vi "Old Vision Processing.vi"(4 "error in (no error)":errorcluster) -> ()   [LabVIEW 2011]
doc: "This VI runs in parallel to other tasks. It gets images from the camera, processes them for color or shape and use that information to affect robot behavior."
uses:
  Robot Global Data.vi
panel:
  out "deltay":dbl
  out "deltax":dbl
  out "distance":dbl
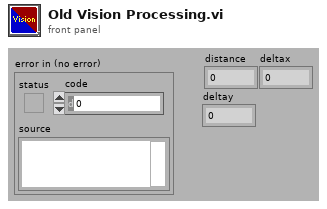
[diagram p1: front panel]
types:
  T1 = typedef "Image Type" = u32
  T2 = typedef "IMAQ Image.ctl" = refnum<image>
  T3 = typedef "WPI_CameraDevRef.ctl" = cluster{"Camera Address":string, "CameraStatus":errorcluster, "Acquire Image Notifier":refnum<notifier>}
  T4 = typedef "WPI_CameraImageSize.ctl" = enum16{"640x480", "320x240", "160x120"}
  T5 = typedef "CAN Data.ctl" = cluster{"Turret Position":dbl, "Turret Elevation":dbl, "Shooter Top Speed":dbl, "Shooter Bottom Speed":dbl}
  T6 = typedef "Position Typedef.ctl" = cluster{"X":dbl, "Y":dbl, "Heading":dbl}
  T7 = typedef "Target Typedef.ctl" = cluster{"X":dbl, "Y":dbl, "Ultrasonic Range (in)":dbl}
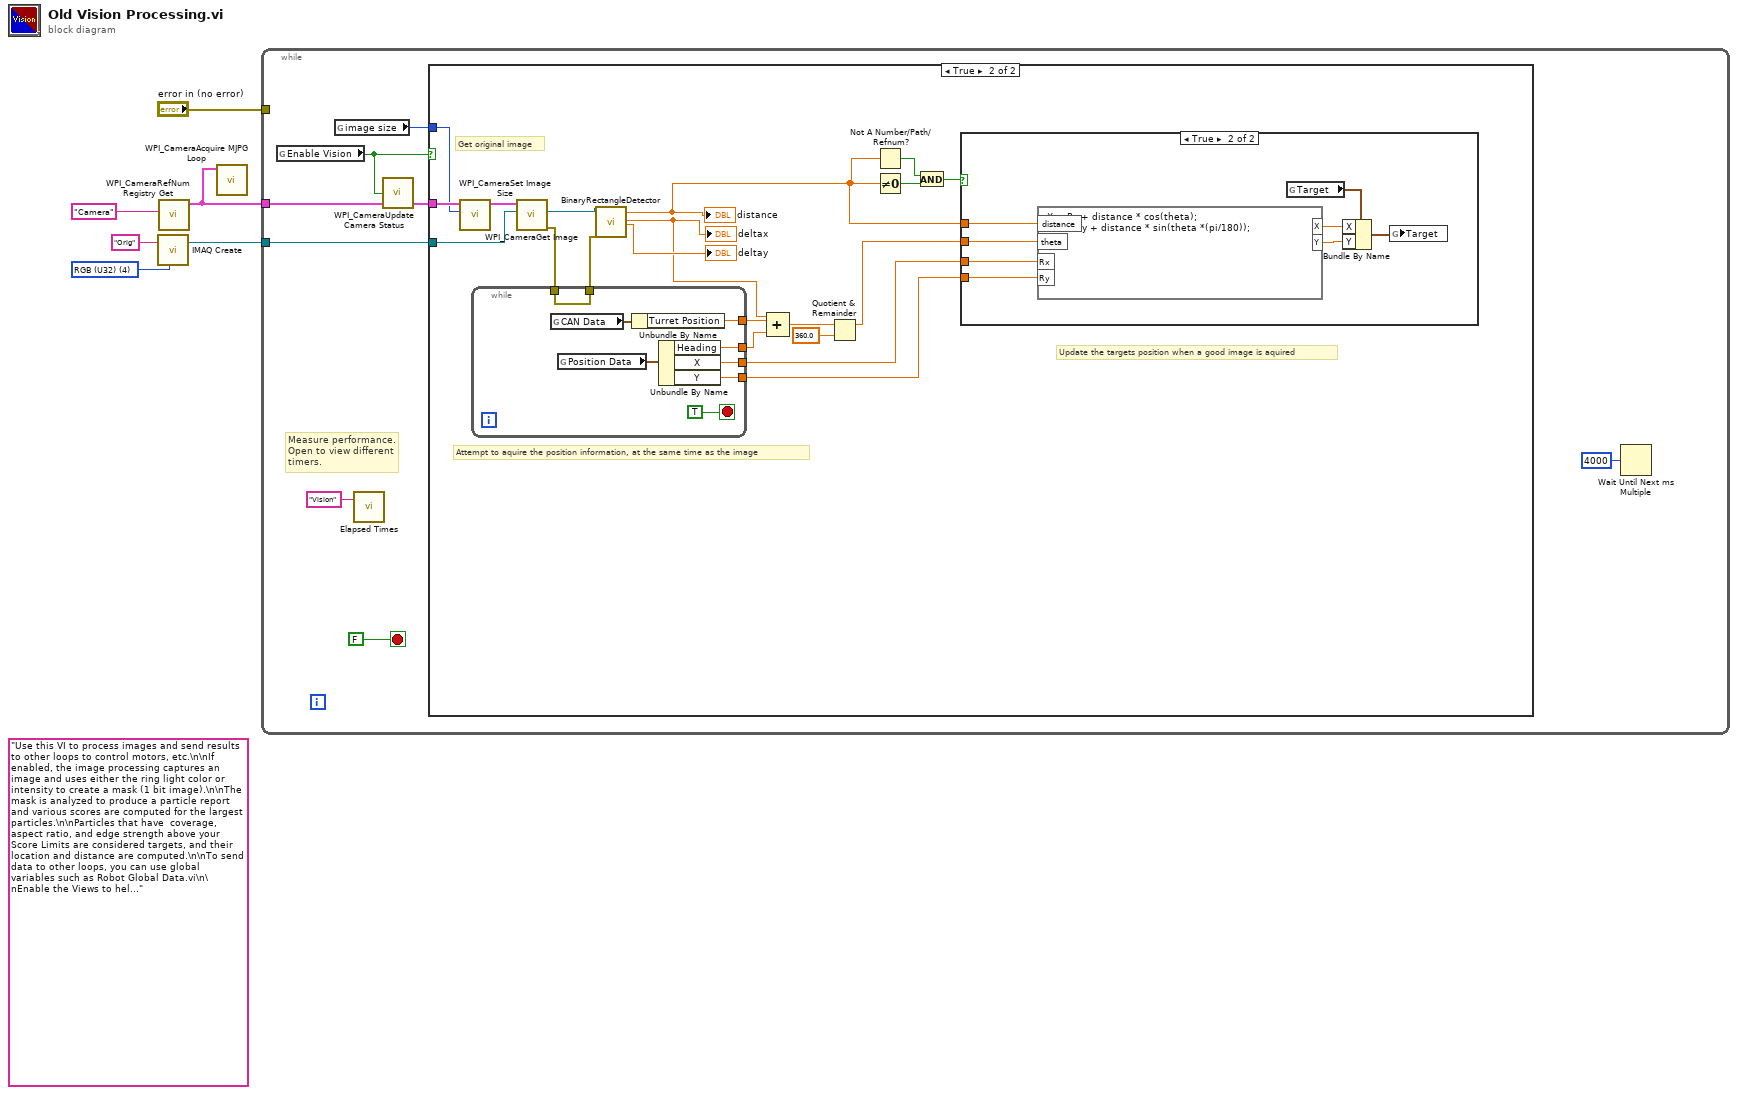
[diagram p0: block diagram]
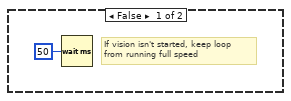
[diagram p2: hidden frame]
diagram:
  w4 = T1 4 items=["Grayscale (U8)", "Grayscale (I16)", "Grayscale (SGL)", "Complex (CSG)", "RGB (U32)", "HSL (U32)", "RGB (U64)", "Grayscale (U16)"] ("Image Type")
  (unwired) "Use this VI to process images and send results to other loops to control motors, etc.\n\nIf enabled, the image processing captures an image and uses either the ring light color or intensity to create a mask (1 bit image).\n\nThe mask is analyzed to produce a particle report and various scores are computed for the largest particles.\n\nParticles that have  coverage, aspect ratio, and edge strength above your Score Limits are considered targets, and their location and distance are computed.\n\nTo send data to other loops, you can use global variables such as Robot Global Data.vi\n\nEnable the Views to help debug color settings. Disable the View to speed up processing."
  n1 = call "IMAQ Create"("Image Name"="Orig", "Image Type"=w4) -> ("New Image"=w3:T2)  [unwired: 2 in, 2 out]
  n2 = call <vilib>:"WPI_CameraRefNum Registry Get.vi"("refnum name"="Camera") -> ("CameraDevRef"=w1:T3)  [unwired: 1 in, 9 out]
  n3 = call <vilib>:"WPI_CameraAcquire MJPG Loop.vi"("CameraDevRef"=w1) -> ()  [unwired: 11 in]
  n4 = while {
    tunnel: w3 -> [w13]
    tunnel: w1 -> [w12]
    tunnel: "error in (no error)" -> [_]
    stop <- FALSE stop-if-true
    # "Measure performance.\nOpen to view different\ntimers."
    n5 = global read "Robot Global Data.vi" "Enable Vision"() -> (w10:bool)
    n6 = global read "Robot Global Data.vi" "image size"() -> (w9:T4)
    n7 = call "Elapsed Times.vi"("Call Name"="Vision") -> ()  [unwired: 2 in, 1 out]
    n8 = call <vilib>:"WPI_CameraUpdate Camera Status.vi"("CameraDevRef In"=w12, "Enable Vision"=w10) -> ("CameraDevRef Out"=w11:T3)  [unwired: 3 in]
    n9 = case shown="True" w10 {
      tunnel: w13 -> [_ w35]
      tunnel: w11 -> [_ w34]
      tunnel: w9 -> [_ w33]
      frame False {
        # "If vision isn't started, keep loop\nfrom running full speed"
        n10 = Wait (ms)(milliseconds to wait=u32 50) -> ()  [unwired: 1 out]
      }
      frame True {
        # "Attempt to aquire the position information, at the same time as the image"
        # "Update the targets position when a good image is aquired"
        # "Get original image"
        n11 = call <vilib>:"WPI_CameraSet Image Size.vi"("Image Size"=w33, "CameraDevRef"=w34) -> ("CameraDevRef Out"=w32:T3)  [unwired: 8 in, 1 out]
        n12 = call <vilib>:"WPI_CameraGet Image.vi"("Image"=w35, "CameraDevRef"=w32) -> ("error out"=w30:errorcluster, "Image Out"=w23:T2)  [unwired: 7 in, 1 out]
        n13 = while {
          tunnel: [w50] -> w28
          tunnel: [w49] -> w22
          tunnel: w30 -> [w49]
          tunnel: [w46] -> w29
          tunnel: [w45] -> w26
          tunnel: [w44] -> w25
          stop <- TRUE stop-if-true
          n14 = global read "Robot Global Data.vi" "CAN Data"() -> (w47:T5)
          n15 = global read "Robot Global Data.vi" "Position Data"() -> (w51:T6)
          n16 = Unbundle By Name(w47) -> ("Turret Position"=w46:dbl)
          n17 = Unbundle By Name(w51) -> ("Heading"=w50:dbl, "X"=w45:dbl, "Y"=w44:dbl)
        }
        n18 = call "BinaryRectangleDetector.vi"("Image In"=w23, "error in"=w22) -> ("distance"=w19:dbl, "deltax"=w20:dbl, "deltay"=→"deltay":dbl)  [unwired: 20 in, 3 out]
        "distance" <- w19
        "deltax" <- w20
        n19 = Compound Arithmetic op=ADD(w20, w29, w28) -> (w31:dbl)
        n20 = Quotient & Remainder(x=w31, y=360.0) -> (x-y*floor(x/y)=w27:dbl)  [unwired: 1 out]
        n21 = Not A Number/Path/Refnum?(number/path/refnum=w19) -> (NaN/Path/Refnum?=w16:bool)
        n22 = Not Equal To 0?(x=w19) -> (x != 0?=w17:bool)
        n23 = And(x=w16, y=w17) -> (x .and. y?=w18:bool)
        n24 = case shown="True" w18 {
          tunnel: w27 -> [_ w39]
          tunnel: w26 -> [_ w38]
          tunnel: w25 -> [_ w37]
          tunnel: w19 -> [_ w36]
          frame False {
          }
          frame True {
            n25 = formula code="X = Rx + distance * cos(theta);\n   Y = Ry + distance * sin(theta *(pi/180));"("Rx"=w38, "Ry"=w37, "distance"=w36, "theta"=w39) -> ("X"=w42:dbl, "Y"=w41:dbl)
            n26 = global read "Robot Global Data.vi" "Target"() -> (w43:T7)
            n27 = Bundle By Name(cluster=w43, "X"=w42, "Y"=w41) -> (w40:T7)
            n28 = global write "Robot Global Data.vi" "Target"(w40) -> ()
          }
        }
      }
    }
    n29 = Wait Until Next ms Multiple(millisecond multiple=u32 4000) -> ()  [unwired: 1 out]
  }
